vi "Mutate System Definition.vi"(8 "error in (no error)":errorcluster, 11 "Device Ref in":T1 format="%.0x") -> (0 "error out":errorcluster, 3 "Device Ref out":T1 format="%.0x")   [LabVIEW 2020, in "Ballard ARINC 429 System Explorer.lvlib" / "Implementation.lvlib"]
uses:
  Implementation.lvlib
  <vilib>/NI VeriStand/Custom Device API/Custom Device Item Ref.ctl
  <vilib>/NI VeriStand/Custom Device API/Custom Device API.lvlib
  Scripting/Ballard/Ballard ARINC 429 Scripting.lvlib
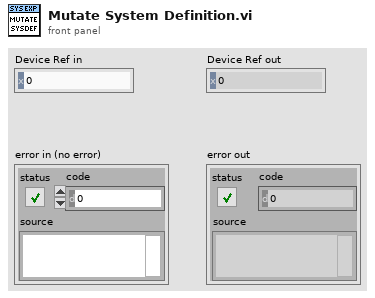
[diagram p1: front panel]
types:
  T1 = typedef "Custom Device API.lvlib/Custom Device Item Ref.ctl" = u64
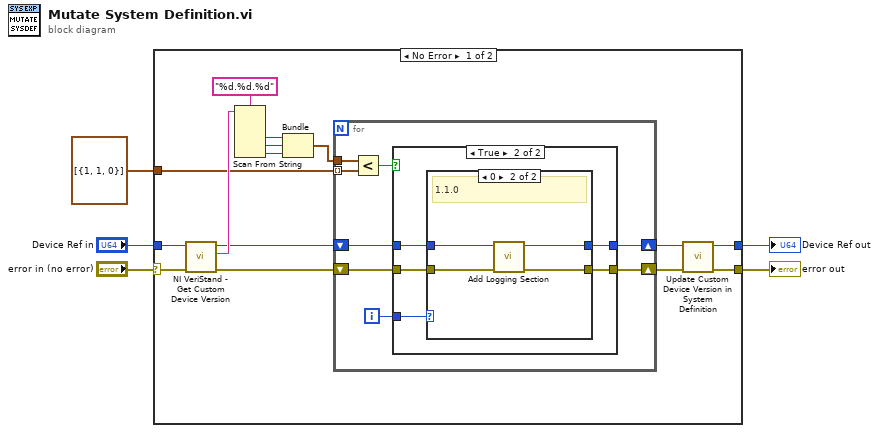
[diagram p0: block diagram]
diagram:
  n1 = case shown="No Error" "error in (no error)" {
    selector: "error in (no error)" -> [w20 w43]
    tunnel: [w6 w43] -> w4
    tunnel: [w7 w42] -> w3
    tunnel: "Device Ref in" -> [w19 w42]
    tunnel: cluster{i32, i32, i32}[] [{1, 1, 0}] ("Array") -> [w10 _]
    frame No Error {
      n2 = call <vilib>:"NI VeriStand - Get Custom Device Version.vi"("error in (no error)"=w20, "Device Ref in"=w19) -> ("error out"=w12:errorcluster, "Value"=w14:string, "Device Ref out"=w11:T1)  [unwired: 7 in]
      n3 = Scan From String(format string="%d.%d.%d", input string=w14) -> (output 1=w17:i32, output 2=w16:i32, output 3=w15:i32)  [unwired: 5 in, 3 out]
      n4 = Bundle(w17, w16, w15) -> (w13:cluster{i32, i32, i32})  [unwired: 1 in]
      n5 = for {
        tunnel: w10 -> [w27] mode=indexing
        tunnel: w13 -> [w28]
        shift-right: [w22] -> w9
        shift-left: w11 -> [w23]
        shift-right: [w25] -> w8
        shift-left: w12 -> [w24]
        i -> [w21]
        n6 = Less?(x=w28, y=w27) -> (x < y?=w26:bool)
        n7 = case shown="True" w26 {
          tunnel: [w29 w34] -> w25
          tunnel: w24 -> [w29 w33]
          tunnel: w23 -> [w30 w31]
          tunnel: [w30 w32] -> w22
          tunnel: w21 -> [_ w35]
          frame False {
          }
          frame True {
            n8 = case shown="0" w35 {
              tunnel: [w36 w40] -> w34
              tunnel: w33 -> [w36 w41]
              tunnel: [w37 w38] -> w32
              tunnel: w31 -> [w37 w39]
              frame Default {
              }
              frame 0 {
                # "1.1.0"
                n9 = call "Add Logging Section.vi"("error in"=w41, "Ballard ARINC 429 custom device in"=w39) -> ("error out"=w40:errorcluster, "Ballard ARINC 429 custom device out"=w38:T1)  [unwired: 7 in, 1 out]
              }
            }
          }
        }
      }
      n10 = call "Update Custom Device Version in System Definition.vi"("error in (no error)"=w8, "Device Ref in"=w9) -> ("error out"=w6:errorcluster, "Device Ref out"=w7:T1)  [unwired: 8 in]
    }
    frame Error {
    }
  }
  "error out" <- w4
  "Device Ref out" <- w3
